vi "Get Loop Parameters.vi"(11 "error in (no error)":errorcluster) -> (4 "Sequence Type":T1, 6 "90Deg Pulse Sequence Array":T11[](array[typedef])=[{"Delay Settings"={"Delay d1"=100.0, "Delay d2"=2.0, "d1 Unit"=0, "d2 Unit"=0}, "Preliminary Settings"={"Nº of Scans (ns)"=3, "Pulse Frequency"=10000000.0}, "Pulse Settings"={"Duration Signal P1"=10.0, "Power Level"=1000, "Phase"=90, "P1 Units"=0}, "Acquisition Settings"={"Number Samples"=5000, "Time Between Points"=0.0, "Unit"=0}}, {"Delay Settings"={"Delay d1"=100.0, "Delay d2"=2.0, "d1 Unit"=0, "d2 Unit"=0}, "Preliminary Settings"={"Nº of Scans (ns)"=3, "Pulse Frequency"=10000000.0}, "Pulse Settings"={"Duration Signal P1"=20.0, "Power Level"=1000, "Phase"=90, "P1 Units"=0}, "Acquisition Settings"={"Number Samples"=5000, "Time Between Points"=0.0, "Unit"=0}}, {"Delay Settings"={"Delay d1"=100.0, "Delay d2"=2.0, "d1 Unit"=0, "d2 Unit"=0}, "Preliminary Settings"={"Nº of Scans (ns)"=3, "Pulse Frequency"=10000000.0}, "Pulse Settings"={"Duration Signal P1"=30.0, "Power Level"=1000, "Phase"=90, "P1 Units"=0}, "Acquisition Settings"={"Number Samples"=5000, "Time Between Points"=0.0, "Unit"=0}}, {"Delay Settings"={"Delay d1"=100.0, "Delay d2"=2.0, "d1 Unit"=0, "d2 Unit"=0}, "Preliminary Settings"={"Nº of Scans (ns)"=3, "Pulse Frequency"=10000000.0}, "Pulse Settings"={"Duration Signal P1"=40.0, "Power Level"=1000, "Phase"=90, "P1 Units"=0}, "Acquisition Settings"={"Number Samples"=5000, "Time Between Points"=0.0, "Unit"=0}}, {"Delay Settings"={"Delay d1"=100.0, "Delay d2"=2.0, "d1 Unit"=0, "d2 Unit"=0}, "Preliminary Settings"={"Nº of Scans (ns)"=3, "Pulse Frequency"=10000000.0}, "Pulse Settings"={"Duration Signal P1"=50.0, "Power Level"=1000, "Phase"=90, "P1 Units"=0}, "Acquisition Settings"={"Number Samples"=5000, "Time Between Points"=0.0, "Unit"=0}}, {"Delay Settings"={"Delay d1"=100.0, "Delay d2"=2.0, "d1 Unit"=0, "d2 Unit"=0}, "Preliminary Settings"={"Nº of Scans (ns)"=3, "Pulse Frequency"=10000000.0}, "Pulse Settings"={"Duration Signal P1"=60.0, "Power Level"=1000, "Phase"=90, "P1 Units"=0}, "Acquisition Settings"={"Number Samples"=5000, "Time Between Points"=0.0, "Unit"=0}}, {"Delay Settings"={"Delay d1"=100.0, "Delay d2"=2.0, "d1 Unit"=0, "d2 Unit"=0}, "Preliminary Settings"={"Nº of Scans (ns)"=3, "Pulse Frequency"=10000000.0}, "Pulse Settings"={"Duration Signal P1"=80.0, "Power Level"=1000, "Phase"=90, "P1 Units"=0}, "Acquisition Settings"={"Number Samples"=5000, "Time Between Points"=0.0, "Unit"=0}}, {"Delay Settings"={"Delay d1"=100.0, "Delay d2"=2.0, "d1 Unit"=0, "d2 Unit"=0}, "Preliminary Settings"={"Nº of Scans (ns)"=3, "Pulse Frequency"=10000000.0}, "Pulse Settings"={"Duration Signal P1"=90.0, "Power Level"=1000, "Phase"=90, "P1 Units"=0}, "Acquisition Settings"={"Number Samples"=5000, "Time Between Points"=0.0, "Unit"=0}}, {"Delay Settings"={"Delay d1"=100.0, "Delay d2"=2.0, "d1 Unit"=0, "d2 Unit"=0}, "Preliminary Settings"={"Nº of Scans (ns)"=3, "Pulse Frequency"=10000000.0}, "Pulse Settings"={"Duration Signal P1"=100.0, "Power Level"=1000, "Phase"=90, "P1 Units"=0}, "Acquisition Settings"={"Number Samples"=5000, "Time Between Points"=0.0, "Unit"=0}}, {"Delay Settings"={"Delay d1"=100.0, "Delay d2"=2.0, "d1 Unit"=0, "d2 Unit"=0}, "Preliminary Settings"={"Nº of Scans (ns)"=3, "Pulse Frequency"=9000000.0}, "Pulse Settings"={"Duration Signal P1"=10.0, "Power Level"=1000, "Phase"=90, "P1 Units"=0}, "Acquisition Settings"={"Number Samples"=5000, "Time Between Points"=0.0, "Unit"=0}}, {"Delay Settings"={"Delay d1"=100.0, "Delay d2"=2.0, "d1 Unit"=0, "d2 Unit"=0}, "Preliminary Settings"={"Nº of Scans (ns)"=3, "Pulse Frequency"=9000000.0}, "Pulse Settings"={"Duration Signal P1"=20.0, "Power Level"=1000, "Phase"=90, "P1 Units"=0}, "Acquisition Settings"={"Number Samples"=5000, "Time Between Points"=0.0, "Unit"=0}}, {"Delay Settings"={"Delay d1"=100.0, "Delay d2"=2.0, "d1 Unit"=0, "d2 Unit"=0}, "Preliminary Settings"={"Nº of Scans (ns)"=3, "Pulse Frequency"=9000000.0}, "Pulse Settings"={"Duration Signal P1"=30.0, "Power Level"=1000, "Phase"=90, "P1 Units"=0}, "Acquisition Settings"={"Number Samples"=5000, "Time Between Points"=0.0, "Unit"=0}}, {"Delay Settings"={"Delay d1"=100.0, "Delay d2"=2.0, "d1 Unit"=0, "d2 Unit"=0}, "Preliminary Settings"={"Nº of Scans (ns)"=3, "Pulse Frequency"=9000000.0}, "Pulse Settings"={"Duration Signal P1"=40.0, "Power Level"=1000, "Phase"=90, "P1 Units"=0}, "Acquisition Settings"={"Number Samples"=5000, "Time Between Points"=0.0, "Unit"=0}}, {"Delay Settings"={"Delay d1"=100.0, "Delay d2"=2.0, "d1 Unit"=0, "d2 Unit"=0}, "Preliminary Settings"={"Nº of Scans (ns)"=3, "Pulse Frequency"=9000000.0}, "Pulse Settings"={"Duration Signal P1"=50.0, "Power Level"=1000, "Phase"=90, "P1 Units"=0}, "Acquisition Settings"={"Number Samples"=5000, "Time Between Points"=0.0, "Unit"=0}}, {"Delay Settings"={"Delay d1"=100.0, "Delay d2"=2.0, "d1 Unit"=0, "d2 Unit"=0}, "Preliminary Settings"={"Nº of Scans (ns)"=3, "Pulse Frequency"=9000000.0}, "Pulse Settings"={"Duration Signal P1"=60.0, "Power Level"=1000, "Phase"=90, "P1 Units"=0}, "Acquisition Settings"={"Number Samples"=5000, "Time Between Points"=0.0, "Unit"=0}}, {"Delay Settings"={"Delay d1"=100.0, "Delay d2"=2.0, "d1 Unit"=0, "d2 Unit"=0}, "Preliminary Settings"={"Nº of Scans (ns)"=3, "Pulse Frequency"=9000000.0}, "Pulse Settings"={"Duration Signal P1"=80.0, "Power Level"=1000, "Phase"=90, "P1 Units"=0}, "Acquisition Settings"={"Number Samples"=5000, "Time Between Points"=0.0, "Unit"=0}}, {"Delay Settings"={"Delay d1"=100.0, "Delay d2"=2.0, "d1 Unit"=0, "d2 Unit"=0}, "Preliminary Settings"={"Nº of Scans (ns)"=3, "Pulse Frequency"=9000000.0}, "Pulse Settings"={"Duration Signal P1"=90.0, "Power Level"=1000, "Phase"=90, "P1 Units"=0}, "Acquisition Settings"={"Number Samples"=5000, "Time Between Points"=0.0, "Unit"=0}}, {"Delay Settings"={"Delay d1"=100.0, "Delay d2"=2.0, "d1 Unit"=0, "d2 Unit"=0}, "Preliminary Settings"={"Nº of Scans (ns)"=3, "Pulse Frequency"=9000000.0}, "Pulse Settings"={"Duration Signal P1"=100.0, "Power Level"=1000, "Phase"=90, "P1 Units"=0}, "Acquisition Settings"={"Number Samples"=5000, "Time Between Points"=0.0, "Unit"=0}}] {"Acquisition Settings"."Unit" items=["us", "ms"]; "Acquisition Settings"."Time Between Points" min=0.0 step=1.0; "Acquisition Settings"."Number Samples" step=1; "Pulse Settings"."P1 Units" items=["us", "ms"]; "Pulse Settings"."Phase" max=270 step=90; "Pulse Settings"."Power Level" max=1023 step=1; "Pulse Settings"."Duration Signal P1" min=0.0 step=1.0 format="%#_4g"; "Preliminary Settings"."Pulse Frequency" min=1.0 max=200000000.0 step=1000000.0 format="%^#_6e"; "Preliminary Settings"."Nº of Scans (ns)" step=1; "Delay Settings"."d2 Unit" items=["us", "ms"]; "Delay Settings"."d1 Unit" items=["us", "ms"]; "Delay Settings"."Delay d2" min=0.0 step=1.0 format="%#_4g"; "Delay Settings"."Delay d1" min=0.0 step=1.0 format="%#_4g"}, 8 "CPMG Pulse Sequence Array":T7[](array[typedef])=[{"Acquisition Settings"={"Number Samples"=5000, "Time Between Points"=0.0, "Unit"=0}, "Delay Settings"={"Delay d1"=100.0, "Delay d2"=2.0, "d1 Unit"=0, "d2 Unit"=0, "Delay d3"=100.0, "d3 Unit"=0, "Delay d4"=2.0, "d4 Unit"=0}, "Preliminary Settings"={"Nº of Scans (ns)"=3, "Pulse Frequency"=10000000.0, "Nº of Echoes (ne)"=3}, "Pulse Settings"={"Duration Signal P1"=10.0, "Power Level P1"=1000, "Phase P1"=90, "P1 Unit"=0, "Duration Signal P2"=10.0, "Power Level P2"=1000, "Phase P2"=90, "P2 Unit"=0}}, {"Acquisition Settings"={"Number Samples"=5000, "Time Between Points"=0.0, "Unit"=0}, "Delay Settings"={"Delay d1"=100.0, "Delay d2"=2.0, "d1 Unit"=0, "d2 Unit"=0, "Delay d3"=100.0, "d3 Unit"=0, "Delay d4"=2.0, "d4 Unit"=0}, "Preliminary Settings"={"Nº of Scans (ns)"=3, "Pulse Frequency"=10000000.0, "Nº of Echoes (ne)"=3}, "Pulse Settings"={"Duration Signal P1"=20.0, "Power Level P1"=1000, "Phase P1"=90, "P1 Unit"=0, "Duration Signal P2"=20.0, "Power Level P2"=1000, "Phase P2"=90, "P2 Unit"=0}}, {"Acquisition Settings"={"Number Samples"=5000, "Time Between Points"=0.0, "Unit"=0}, "Delay Settings"={"Delay d1"=100.0, "Delay d2"=2.0, "d1 Unit"=0, "d2 Unit"=0, "Delay d3"=100.0, "d3 Unit"=0, "Delay d4"=2.0, "d4 Unit"=0}, "Preliminary Settings"={"Nº of Scans (ns)"=3, "Pulse Frequency"=10000000.0, "Nº of Echoes (ne)"=3}, "Pulse Settings"={"Duration Signal P1"=30.0, "Power Level P1"=1000, "Phase P1"=90, "P1 Unit"=0, "Duration Signal P2"=30.0, "Power Level P2"=1000, "Phase P2"=90, "P2 Unit"=0}}, {"Acquisition Settings"={"Number Samples"=5000, "Time Between Points"=0.0, "Unit"=0}, "Delay Settings"={"Delay d1"=100.0, "Delay d2"=2.0, "d1 Unit"=0, "d2 Unit"=0, "Delay d3"=100.0, "d3 Unit"=0, "Delay d4"=2.0, "d4 Unit"=0}, "Preliminary Settings"={"Nº of Scans (ns)"=3, "Pulse Frequency"=10000000.0, "Nº of Echoes (ne)"=3}, "Pulse Settings"={"Duration Signal P1"=40.0, "Power Level P1"=1000, "Phase P1"=90, "P1 Unit"=0, "Duration Signal P2"=40.0, "Power Level P2"=1000, "Phase P2"=90, "P2 Unit"=0}}, {"Acquisition Settings"={"Number Samples"=5000, "Time Between Points"=0.0, "Unit"=0}, "Delay Settings"={"Delay d1"=100.0, "Delay d2"=2.0, "d1 Unit"=0, "d2 Unit"=0, "Delay d3"=100.0, "d3 Unit"=0, "Delay d4"=2.0, "d4 Unit"=0}, "Preliminary Settings"={"Nº of Scans (ns)"=3, "Pulse Frequency"=10000000.0, "Nº of Echoes (ne)"=3}, "Pulse Settings"={"Duration Signal P1"=50.0, "Power Level P1"=1000, "Phase P1"=90, "P1 Unit"=0, "Duration Signal P2"=50.0, "Power Level P2"=1000, "Phase P2"=90, "P2 Unit"=0}}, {"Acquisition Settings"={"Number Samples"=5000, "Time Between Points"=0.0, "Unit"=0}, "Delay Settings"={"Delay d1"=100.0, "Delay d2"=2.0, "d1 Unit"=0, "d2 Unit"=0, "Delay d3"=100.0, "d3 Unit"=0, "Delay d4"=2.0, "d4 Unit"=0}, "Preliminary Settings"={"Nº of Scans (ns)"=3, "Pulse Frequency"=10000000.0, "Nº of Echoes (ne)"=3}, "Pulse Settings"={"Duration Signal P1"=60.0, "Power Level P1"=1000, "Phase P1"=90, "P1 Unit"=0, "Duration Signal P2"=60.0, "Power Level P2"=1000, "Phase P2"=90, "P2 Unit"=0}}, {"Acquisition Settings"={"Number Samples"=5000, "Time Between Points"=0.0, "Unit"=0}, "Delay Settings"={"Delay d1"=100.0, "Delay d2"=2.0, "d1 Unit"=0, "d2 Unit"=0, "Delay d3"=100.0, "d3 Unit"=0, "Delay d4"=2.0, "d4 Unit"=0}, "Preliminary Settings"={"Nº of Scans (ns)"=3, "Pulse Frequency"=10000000.0, "Nº of Echoes (ne)"=3}, "Pulse Settings"={"Duration Signal P1"=80.0, "Power Level P1"=1000, "Phase P1"=90, "P1 Unit"=0, "Duration Signal P2"=80.0, "Power Level P2"=1000, "Phase P2"=90, "P2 Unit"=0}}, {"Acquisition Settings"={"Number Samples"=5000, "Time Between Points"=0.0, "Unit"=0}, "Delay Settings"={"Delay d1"=100.0, "Delay d2"=2.0, "d1 Unit"=0, "d2 Unit"=0, "Delay d3"=100.0, "d3 Unit"=0, "Delay d4"=2.0, "d4 Unit"=0}, "Preliminary Settings"={"Nº of Scans (ns)"=3, "Pulse Frequency"=10000000.0, "Nº of Echoes (ne)"=3}, "Pulse Settings"={"Duration Signal P1"=90.0, "Power Level P1"=1000, "Phase P1"=90, "P1 Unit"=0, "Duration Signal P2"=90.0, "Power Level P2"=1000, "Phase P2"=90, "P2 Unit"=0}}, {"Acquisition Settings"={"Number Samples"=5000, "Time Between Points"=0.0, "Unit"=0}, "Delay Settings"={"Delay d1"=100.0, "Delay d2"=2.0, "d1 Unit"=0, "d2 Unit"=0, "Delay d3"=100.0, "d3 Unit"=0, "Delay d4"=2.0, "d4 Unit"=0}, "Preliminary Settings"={"Nº of Scans (ns)"=3, "Pulse Frequency"=10000000.0, "Nº of Echoes (ne)"=3}, "Pulse Settings"={"Duration Signal P1"=100.0, "Power Level P1"=1000, "Phase P1"=90, "P1 Unit"=0, "Duration Signal P2"=100.0, "Power Level P2"=1000, "Phase P2"=90, "P2 Unit"=0}}, {"Acquisition Settings"={"Number Samples"=5000, "Time Between Points"=0.0, "Unit"=0}, "Delay Settings"={"Delay d1"=100.0, "Delay d2"=2.0, "d1 Unit"=0, "d2 Unit"=0, "Delay d3"=100.0, "d3 Unit"=0, "Delay d4"=2.0, "d4 Unit"=0}, "Preliminary Settings"={"Nº of Scans (ns)"=3, "Pulse Frequency"=9000000.0, "Nº of Echoes (ne)"=3}, "Pulse Settings"={"Duration Signal P1"=10.0, "Power Level P1"=1000, "Phase P1"=90, "P1 Unit"=0, "Duration Signal P2"=10.0, "Power Level P2"=1000, "Phase P2"=90, "P2 Unit"=0}}, {"Acquisition Settings"={"Number Samples"=5000, "Time Between Points"=0.0, "Unit"=0}, "Delay Settings"={"Delay d1"=100.0, "Delay d2"=2.0, "d1 Unit"=0, "d2 Unit"=0, "Delay d3"=100.0, "d3 Unit"=0, "Delay d4"=2.0, "d4 Unit"=0}, "Preliminary Settings"={"Nº of Scans (ns)"=3, "Pulse Frequency"=9000000.0, "Nº of Echoes (ne)"=3}, "Pulse Settings"={"Duration Signal P1"=20.0, "Power Level P1"=1000, "Phase P1"=90, "P1 Unit"=0, "Duration Signal P2"=20.0, "Power Level P2"=1000, "Phase P2"=90, "P2 Unit"=0}}, {"Acquisition Settings"={"Number Samples"=5000, "Time Between Points"=0.0, "Unit"=0}, "Delay Settings"={"Delay d1"=100.0, "Delay d2"=2.0, "d1 Unit"=0, "d2 Unit"=0, "Delay d3"=100.0, "d3 Unit"=0, "Delay d4"=2.0, "d4 Unit"=0}, "Preliminary Settings"={"Nº of Scans (ns)"=3, "Pulse Frequency"=9000000.0, "Nº of Echoes (ne)"=3}, "Pulse Settings"={"Duration Signal P1"=30.0, "Power Level P1"=1000, "Phase P1"=90, "P1 Unit"=0, "Duration Signal P2"=30.0, "Power Level P2"=1000, "Phase P2"=90, "P2 Unit"=0}}, {"Acquisition Settings"={"Number Samples"=5000, "Time Between Points"=0.0, "Unit"=0}, "Delay Settings"={"Delay d1"=100.0, "Delay d2"=2.0, "d1 Unit"=0, "d2 Unit"=0, "Delay d3"=100.0, "d3 Unit"=0, "Delay d4"=2.0, "d4 Unit"=0}, "Preliminary Settings"={"Nº of Scans (ns)"=3, "Pulse Frequency"=9000000.0, "Nº of Echoes (ne)"=3}, "Pulse Settings"={"Duration Signal P1"=40.0, "Power Level P1"=1000, "Phase P1"=90, "P1 Unit"=0, "Duration Signal P2"=40.0, "Power Level P2"=1000, "Phase P2"=90, "P2 Unit"=0}}, {"Acquisition Settings"={"Number Samples"=5000, "Time Between Points"=0.0, "Unit"=0}, "Delay Settings"={"Delay d1"=100.0, "Delay d2"=2.0, "d1 Unit"=0, "d2 Unit"=0, "Delay d3"=100.0, "d3 Unit"=0, "Delay d4"=2.0, "d4 Unit"=0}, "Preliminary Settings"={"Nº of Scans (ns)"=3, "Pulse Frequency"=9000000.0, "Nº of Echoes (ne)"=3}, "Pulse Settings"={"Duration Signal P1"=50.0, "Power Level P1"=1000, "Phase P1"=90, "P1 Unit"=0, "Duration Signal P2"=50.0, "Power Level P2"=1000, "Phase P2"=90, "P2 Unit"=0}}, {"Acquisition Settings"={"Number Samples"=5000, "Time Between Points"=0.0, "Unit"=0}, "Delay Settings"={"Delay d1"=100.0, "Delay d2"=2.0, "d1 Unit"=0, "d2 Unit"=0, "Delay d3"=100.0, "d3 Unit"=0, "Delay d4"=2.0, "d4 Unit"=0}, "Preliminary Settings"={"Nº of Scans (ns)"=3, "Pulse Frequency"=9000000.0, "Nº of Echoes (ne)"=3}, "Pulse Settings"={"Duration Signal P1"=60.0, "Power Level P1"=1000, "Phase P1"=90, "P1 Unit"=0, "Duration Signal P2"=60.0, "Power Level P2"=1000, "Phase P2"=90, "P2 Unit"=0}}, {"Acquisition Settings"={"Number Samples"=5000, "Time Between Points"=0.0, "Unit"=0}, "Delay Settings"={"Delay d1"=100.0, "Delay d2"=2.0, "d1 Unit"=0, "d2 Unit"=0, "Delay d3"=100.0, "d3 Unit"=0, "Delay d4"=2.0, "d4 Unit"=0}, "Preliminary Settings"={"Nº of Scans (ns)"=3, "Pulse Frequency"=9000000.0, "Nº of Echoes (ne)"=3}, "Pulse Settings"={"Duration Signal P1"=80.0, "Power Level P1"=1000, "Phase P1"=90, "P1 Unit"=0, "Duration Signal P2"=80.0, "Power Level P2"=1000, "Phase P2"=90, "P2 Unit"=0}}, {"Acquisition Settings"={"Number Samples"=5000, "Time Between Points"=0.0, "Unit"=0}, "Delay Settings"={"Delay d1"=100.0, "Delay d2"=2.0, "d1 Unit"=0, "d2 Unit"=0, "Delay d3"=100.0, "d3 Unit"=0, "Delay d4"=2.0, "d4 Unit"=0}, "Preliminary Settings"={"Nº of Scans (ns)"=3, "Pulse Frequency"=9000000.0, "Nº of Echoes (ne)"=3}, "Pulse Settings"={"Duration Signal P1"=90.0, "Power Level P1"=1000, "Phase P1"=90, "P1 Unit"=0, "Duration Signal P2"=90.0, "Power Level P2"=1000, "Phase P2"=90, "P2 Unit"=0}}, {"Acquisition Settings"={"Number Samples"=5000, "Time Between Points"=0.0, "Unit"=0}, "Delay Settings"={"Delay d1"=100.0, "Delay d2"=2.0, "d1 Unit"=0, "d2 Unit"=0, "Delay d3"=100.0, "d3 Unit"=0, "Delay d4"=2.0, "d4 Unit"=0}, "Preliminary Settings"={"Nº of Scans (ns)"=3, "Pulse Frequency"=9000000.0, "Nº of Echoes (ne)"=3}, "Pulse Settings"={"Duration Signal P1"=100.0, "Power Level P1"=1000, "Phase P1"=90, "P1 Unit"=0, "Duration Signal P2"=100.0, "Power Level P2"=1000, "Phase P2"=90, "P2 Unit"=0}}] {"Pulse Settings"."P2 Unit" items=["us", "ms"]; "Pulse Settings"."Phase P2" max=270 step=90; "Pulse Settings"."Power Level P2" max=1023 step=1; "Pulse Settings"."Duration Signal P2" min=0.0 step=1.0 format="%#_4g"; "Pulse Settings"."P1 Unit" items=["us", "ms"]; "Pulse Settings"."Phase P1" max=270 step=90; "Pulse Settings"."Power Level P1" max=1023 step=1; "Pulse Settings"."Duration Signal P1" min=0.0 step=1.0 format="%#_4g"; "Preliminary Settings"."Nº of Echoes (ne)" step=1; "Preliminary Settings"."Pulse Frequency" min=1.0 max=200000000.0 step=1000000.0 format="%^#_6e"; "Preliminary Settings"."Nº of Scans (ns)" step=1; "Delay Settings"."d4 Unit" items=["us", "ms"]; "Delay Settings"."Delay d4" min=0.0 step=1.0 format="%#_4g"; "Delay Settings"."d3 Unit" items=["us", "ms"]; "Delay Settings"."Delay d3" min=0.0 step=1.0 format="%#_4g"; "Delay Settings"."d2 Unit" items=["us", "ms"]; "Delay Settings"."d1 Unit" items=["us", "ms"]; "Delay Settings"."Delay d2" min=0.0 step=1.0 format="%#_4g"; "Delay Settings"."Delay d1" min=0.0 step=1.0 format="%#_4g"; "Acquisition Settings"."Unit" items=["us", "ms"]; "Acquisition Settings"."Time Between Points" min=0.0 step=1.0; "Acquisition Settings"."Number Samples" step=1}, 10 "T1 Pulse Sequence Array":T2[](array[typedef])=[{"Preliminary Settings"={"Nº of Scans (ns)"=3, "Pulse Frequency"=10000000.0, "Nº of Vd"=3}, "Pulse Settings"={"Duration Signal P2"=10.0, "Power Level P2"=1000, "Phase P2"=90, "P2 Unit"=0, "Duration Signal P1"=10.0, "Power Level P1"=1000, "Phase P1"=90, "P1 Unit"=0}, "Acquisition Settings"={"Number Samples"=5000, "Time Between Points"=0.0, "Unit"=0}, "Delay Settings"={"Delay d1"=100.0, "Delay d2"=2.0, "d1 Unit"=0, "d2 Unit"=0, "Delay d30"=0.0, "d30 Unit"=0, "Vd Unit"=0, "Vd Values"="Automatic"}}, {"Preliminary Settings"={"Nº of Scans (ns)"=3, "Pulse Frequency"=10000000.0, "Nº of Vd"=3}, "Pulse Settings"={"Duration Signal P2"=20.0, "Power Level P2"=1000, "Phase P2"=90, "P2 Unit"=0, "Duration Signal P1"=20.0, "Power Level P1"=1000, "Phase P1"=90, "P1 Unit"=0}, "Acquisition Settings"={"Number Samples"=5000, "Time Between Points"=0.0, "Unit"=0}, "Delay Settings"={"Delay d1"=100.0, "Delay d2"=2.0, "d1 Unit"=0, "d2 Unit"=0, "Delay d30"=0.0, "d30 Unit"=0, "Vd Unit"=0, "Vd Values"="Automatic"}}, {"Preliminary Settings"={"Nº of Scans (ns)"=3, "Pulse Frequency"=10000000.0, "Nº of Vd"=3}, "Pulse Settings"={"Duration Signal P2"=30.0, "Power Level P2"=1000, "Phase P2"=90, "P2 Unit"=0, "Duration Signal P1"=30.0, "Power Level P1"=1000, "Phase P1"=90, "P1 Unit"=0}, "Acquisition Settings"={"Number Samples"=5000, "Time Between Points"=0.0, "Unit"=0}, "Delay Settings"={"Delay d1"=100.0, "Delay d2"=2.0, "d1 Unit"=0, "d2 Unit"=0, "Delay d30"=0.0, "d30 Unit"=0, "Vd Unit"=0, "Vd Values"="Automatic"}}, {"Preliminary Settings"={"Nº of Scans (ns)"=3, "Pulse Frequency"=10000000.0, "Nº of Vd"=3}, "Pulse Settings"={"Duration Signal P2"=40.0, "Power Level P2"=1000, "Phase P2"=90, "P2 Unit"=0, "Duration Signal P1"=40.0, "Power Level P1"=1000, "Phase P1"=90, "P1 Unit"=0}, "Acquisition Settings"={"Number Samples"=5000, "Time Between Points"=1.0, "Unit"=0}, "Delay Settings"={"Delay d1"=100.0, "Delay d2"=2.0, "d1 Unit"=0, "d2 Unit"=0, "Delay d30"=0.0, "d30 Unit"=0, "Vd Unit"=0, "Vd Values"="Automatic"}}, {"Preliminary Settings"={"Nº of Scans (ns)"=3, "Pulse Frequency"=10000000.0, "Nº of Vd"=3}, "Pulse Settings"={"Duration Signal P2"=50.0, "Power Level P2"=1000, "Phase P2"=90, "P2 Unit"=0, "Duration Signal P1"=50.0, "Power Level P1"=1000, "Phase P1"=90, "P1 Unit"=0}, "Acquisition Settings"={"Number Samples"=5000, "Time Between Points"=0.0, "Unit"=0}, "Delay Settings"={"Delay d1"=100.0, "Delay d2"=2.0, "d1 Unit"=0, "d2 Unit"=0, "Delay d30"=0.0, "d30 Unit"=0, "Vd Unit"=0, "Vd Values"="Automatic"}}, {"Preliminary Settings"={"Nº of Scans (ns)"=3, "Pulse Frequency"=10000000.0, "Nº of Vd"=3}, "Pulse Settings"={"Duration Signal P2"=60.0, "Power Level P2"=1000, "Phase P2"=90, "P2 Unit"=0, "Duration Signal P1"=60.0, "Power Level P1"=1000, "Phase P1"=90, "P1 Unit"=0}, "Acquisition Settings"={"Number Samples"=5000, "Time Between Points"=0.0, "Unit"=0}, "Delay Settings"={"Delay d1"=100.0, "Delay d2"=2.0, "d1 Unit"=0, "d2 Unit"=0, "Delay d30"=0.0, "d30 Unit"=0, "Vd Unit"=0, "Vd Values"="Automatic"}}, {"Preliminary Settings"={"Nº of Scans (ns)"=3, "Pulse Frequency"=10000000.0, "Nº of Vd"=3}, "Pulse Settings"={"Duration Signal P2"=80.0, "Power Level P2"=1000, "Phase P2"=90, "P2 Unit"=0, "Duration Signal P1"=80.0, "Power Level P1"=1000, "Phase P1"=90, "P1 Unit"=0}, "Acquisition Settings"={"Number Samples"=5000, "Time Between Points"=1.0, "Unit"=0}, "Delay Settings"={"Delay d1"=100.0, "Delay d2"=2.0, "d1 Unit"=0, "d2 Unit"=0, "Delay d30"=0.0, "d30 Unit"=0, "Vd Unit"=0, "Vd Values"="Automatic"}}, {"Preliminary Settings"={"Nº of Scans (ns)"=3, "Pulse Frequency"=10000000.0, "Nº of Vd"=3}, "Pulse Settings"={"Duration Signal P2"=90.0, "Power Level P2"=1000, "Phase P2"=90, "P2 Unit"=0, "Duration Signal P1"=90.0, "Power Level P1"=1000, "Phase P1"=90, "P1 Unit"=0}, "Acquisition Settings"={"Number Samples"=5000, "Time Between Points"=0.0, "Unit"=0}, "Delay Settings"={"Delay d1"=100.0, "Delay d2"=2.0, "d1 Unit"=0, "d2 Unit"=0, "Delay d30"=0.0, "d30 Unit"=0, "Vd Unit"=0, "Vd Values"="Automatic"}}, {"Preliminary Settings"={"Nº of Scans (ns)"=3, "Pulse Frequency"=10000000.0, "Nº of Vd"=3}, "Pulse Settings"={"Duration Signal P2"=100.0, "Power Level P2"=1000, "Phase P2"=90, "P2 Unit"=0, "Duration Signal P1"=100.0, "Power Level P1"=1000, "Phase P1"=90, "P1 Unit"=0}, "Acquisition Settings"={"Number Samples"=5000, "Time Between Points"=1.0, "Unit"=0}, "Delay Settings"={"Delay d1"=100.0, "Delay d2"=2.0, "d1 Unit"=0, "d2 Unit"=0, "Delay d30"=0.0, "d30 Unit"=0, "Vd Unit"=0, "Vd Values"="Automatic"}}, {"Preliminary Settings"={"Nº of Scans (ns)"=3, "Pulse Frequency"=9000000.0, "Nº of Vd"=3}, "Pulse Settings"={"Duration Signal P2"=10.0, "Power Level P2"=1000, "Phase P2"=90, "P2 Unit"=0, "Duration Signal P1"=10.0, "Power Level P1"=1000, "Phase P1"=90, "P1 Unit"=0}, "Acquisition Settings"={"Number Samples"=5000, "Time Between Points"=20.0, "Unit"=0}, "Delay Settings"={"Delay d1"=100.0, "Delay d2"=2.0, "d1 Unit"=0, "d2 Unit"=0, "Delay d30"=0.0, "d30 Unit"=0, "Vd Unit"=0, "Vd Values"="Automatic"}}, {"Preliminary Settings"={"Nº of Scans (ns)"=3, "Pulse Frequency"=9000000.0, "Nº of Vd"=3}, "Pulse Settings"={"Duration Signal P2"=20.0, "Power Level P2"=1000, "Phase P2"=90, "P2 Unit"=0, "Duration Signal P1"=20.0, "Power Level P1"=1000, "Phase P1"=90, "P1 Unit"=0}, "Acquisition Settings"={"Number Samples"=5000, "Time Between Points"=0.0, "Unit"=0}, "Delay Settings"={"Delay d1"=100.0, "Delay d2"=2.0, "d1 Unit"=0, "d2 Unit"=0, "Delay d30"=0.0, "d30 Unit"=0, "Vd Unit"=0, "Vd Values"="Automatic"}}, {"Preliminary Settings"={"Nº of Scans (ns)"=3, "Pulse Frequency"=9000000.0, "Nº of Vd"=3}, "Pulse Settings"={"Duration Signal P2"=30.0, "Power Level P2"=1000, "Phase P2"=90, "P2 Unit"=0, "Duration Signal P1"=30.0, "Power Level P1"=1000, "Phase P1"=90, "P1 Unit"=0}, "Acquisition Settings"={"Number Samples"=5000, "Time Between Points"=0.0, "Unit"=0}, "Delay Settings"={"Delay d1"=100.0, "Delay d2"=2.0, "d1 Unit"=0, "d2 Unit"=0, "Delay d30"=0.0, "d30 Unit"=0, "Vd Unit"=0, "Vd Values"="Automatic"}}, {"Preliminary Settings"={"Nº of Scans (ns)"=3, "Pulse Frequency"=9000000.0, "Nº of Vd"=3}, "Pulse Settings"={"Duration Signal P2"=40.0, "Power Level P2"=1000, "Phase P2"=90, "P2 Unit"=0, "Duration Signal P1"=40.0, "Power Level P1"=1000, "Phase P1"=90, "P1 Unit"=0}, "Acquisition Settings"={"Number Samples"=5000, "Time Between Points"=20.0, "Unit"=0}, "Delay Settings"={"Delay d1"=100.0, "Delay d2"=2.0, "d1 Unit"=0, "d2 Unit"=0, "Delay d30"=0.0, "d30 Unit"=0, "Vd Unit"=0, "Vd Values"="Automatic"}}, {"Preliminary Settings"={"Nº of Scans (ns)"=3, "Pulse Frequency"=9000000.0, "Nº of Vd"=3}, "Pulse Settings"={"Duration Signal P2"=50.0, "Power Level P2"=1000, "Phase P2"=90, "P2 Unit"=0, "Duration Signal P1"=50.0, "Power Level P1"=1000, "Phase P1"=90, "P1 Unit"=0}, "Acquisition Settings"={"Number Samples"=5000, "Time Between Points"=0.0, "Unit"=0}, "Delay Settings"={"Delay d1"=100.0, "Delay d2"=2.0, "d1 Unit"=0, "d2 Unit"=0, "Delay d30"=0.0, "d30 Unit"=0, "Vd Unit"=0, "Vd Values"="Automatic"}}, {"Preliminary Settings"={"Nº of Scans (ns)"=3, "Pulse Frequency"=9000000.0, "Nº of Vd"=3}, "Pulse Settings"={"Duration Signal P2"=60.0, "Power Level P2"=1000, "Phase P2"=90, "P2 Unit"=0, "Duration Signal P1"=60.0, "Power Level P1"=1000, "Phase P1"=90, "P1 Unit"=0}, "Acquisition Settings"={"Number Samples"=5000, "Time Between Points"=0.0, "Unit"=0}, "Delay Settings"={"Delay d1"=100.0, "Delay d2"=2.0, "d1 Unit"=0, "d2 Unit"=0, "Delay d30"=0.0, "d30 Unit"=0, "Vd Unit"=0, "Vd Values"="Automatic"}}, {"Preliminary Settings"={"Nº of Scans (ns)"=3, "Pulse Frequency"=9000000.0, "Nº of Vd"=3}, "Pulse Settings"={"Duration Signal P2"=80.0, "Power Level P2"=1000, "Phase P2"=90, "P2 Unit"=0, "Duration Signal P1"=80.0, "Power Level P1"=1000, "Phase P1"=90, "P1 Unit"=0}, "Acquisition Settings"={"Number Samples"=5000, "Time Between Points"=0.0, "Unit"=0}, "Delay Settings"={"Delay d1"=100.0, "Delay d2"=2.0, "d1 Unit"=0, "d2 Unit"=0, "Delay d30"=0.0, "d30 Unit"=0, "Vd Unit"=0, "Vd Values"="Automatic"}}, {"Preliminary Settings"={"Nº of Scans (ns)"=3, "Pulse Frequency"=9000000.0, "Nº of Vd"=3}, "Pulse Settings"={"Duration Signal P2"=90.0, "Power Level P2"=1000, "Phase P2"=90, "P2 Unit"=0, "Duration Signal P1"=90.0, "Power Level P1"=1000, "Phase P1"=90, "P1 Unit"=0}, "Acquisition Settings"={"Number Samples"=5000, "Time Between Points"=20.0, "Unit"=0}, "Delay Settings"={"Delay d1"=100.0, "Delay d2"=2.0, "d1 Unit"=0, "d2 Unit"=0, "Delay d30"=0.0, "d30 Unit"=0, "Vd Unit"=0, "Vd Values"="Automatic"}}, {"Preliminary Settings"={"Nº of Scans (ns)"=3, "Pulse Frequency"=9000000.0, "Nº of Vd"=3}, "Pulse Settings"={"Duration Signal P2"=100.0, "Power Level P2"=1000, "Phase P2"=90, "P2 Unit"=0, "Duration Signal P1"=100.0, "Power Level P1"=1000, "Phase P1"=90, "P1 Unit"=0}, "Acquisition Settings"={"Number Samples"=5000, "Time Between Points"=20.0, "Unit"=0}, "Delay Settings"={"Delay d1"=100.0, "Delay d2"=2.0, "d1 Unit"=0, "d2 Unit"=0, "Delay d30"=0.0, "d30 Unit"=0, "Vd Unit"=0, "Vd Values"="Automatic"}}] {"Delay Settings"."Vd Unit" items=["us", "ms"]; "Delay Settings"."d30 Unit" items=["us", "ms"]; "Delay Settings"."Delay d30" min=0.0 step=1.0; "Delay Settings"."d2 Unit" items=["us", "ms"]; "Delay Settings"."d1 Unit" items=["us", "ms"]; "Delay Settings"."Delay d2" min=0.0 step=1.0 format="%#_4g"; "Delay Settings"."Delay d1" min=0.0 step=1.0 format="%#_4g"; "Acquisition Settings"."Unit" items=["us", "ms"]; "Acquisition Settings"."Time Between Points" min=0.0 step=1.0; "Acquisition Settings"."Number Samples" step=1; "Pulse Settings"."P1 Unit" items=["us", "ms"]; "Pulse Settings"."Phase P1" max=270 step=90; "Pulse Settings"."Power Level P1" max=1023 step=1; "Pulse Settings"."Duration Signal P1" min=0.0 step=1.0 format="%#_4g"; "Pulse Settings"."P2 Unit" items=["us", "ms"]; "Pulse Settings"."Phase P2" max=270 step=90; "Pulse Settings"."Power Level P2" max=1023 step=1; "Pulse Settings"."Duration Signal P2" min=0.0 step=1.0 format="%#_4g"; "Preliminary Settings"."Nº of Vd" step=1; "Preliminary Settings"."Pulse Frequency" min=1.0 max=200000000.0 step=1000000.0 format="%^#_6e"; "Preliminary Settings"."Nº of Scans (ns)" step=1}, 12 "90Deg path array":path[](array[path]), 13 "CPMG Path array":path[](array[path]), 14 "T1 path array":path[](array[path]), 15 "error out":errorcluster)   [LabVIEW 2011]
uses:
  Controls/Full_90 Degree Pulse Settings.ctl
  Controls/90D_Delay Settings.ctl
  Controls/90D_Preliminary Settings.ctl
  Controls/90D_Pulse Settings.ctl
  Controls/Acquisition Settings.ctl
  Controls/Full_CPMG Degree Pulse Settings.ctl
  Controls/CPMG_Delay Settings.ctl
  Controls/CPMG_Preliminary Settings.ctl
  Controls/CPMG_Pulse Settings.ctl
  Controls/Full_T1 Degree Pulse Settings.ctl
  Controls/T1_Preliminary Settings.ctl
  Controls/T1_Pulse Settings.ctl
  Controls/T1_Delay Settings.ctl
  Controls/NMR Pulse Sequence Type.ctl
  <vilib>/Utility/file.llb/Read From Spreadsheet File (string).vi
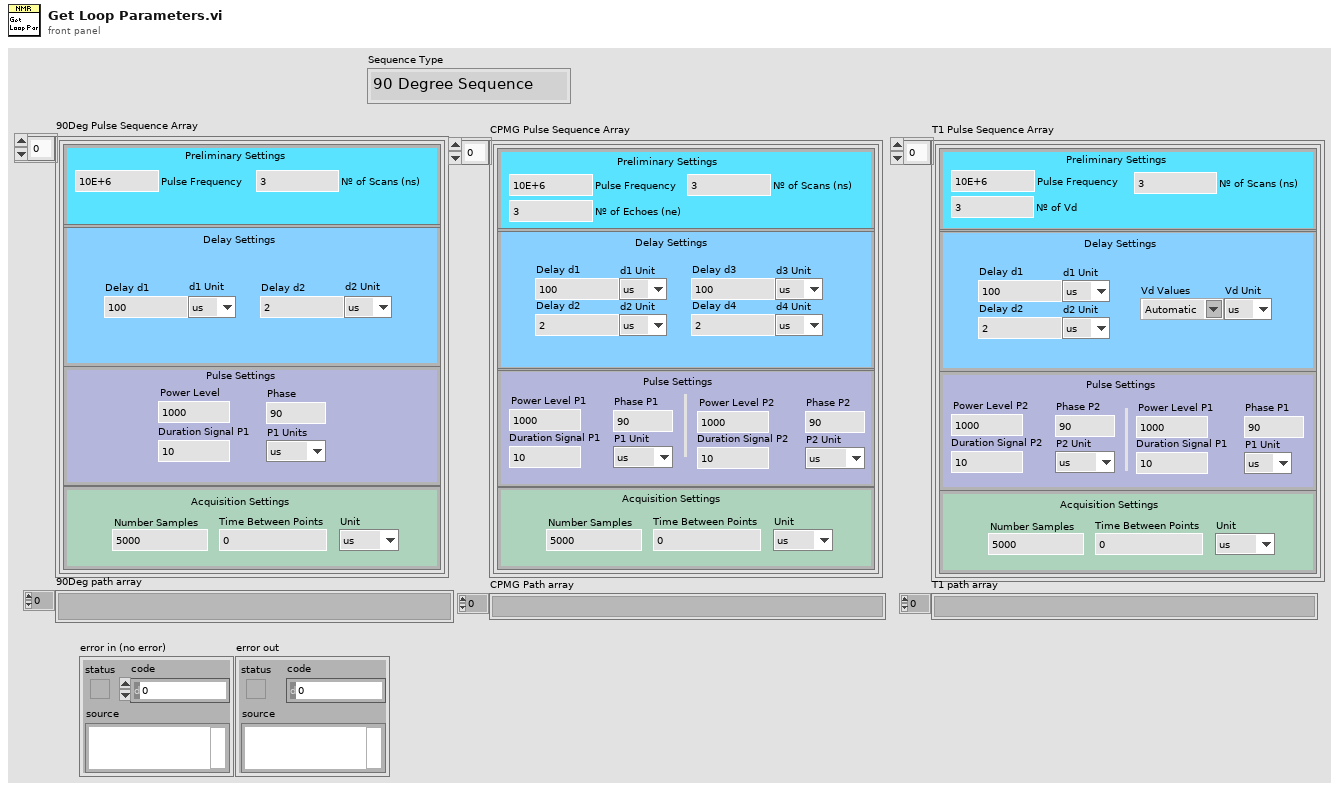
[diagram p1: front panel]
types:
  T1 = typedef "NMR Pulse Sequence Type.ctl" = enum16{"90 Degree Sequence", "CPMG Pulse Sequence", "T1 Pulse Sequence"}
  T2 = typedef "Full_T1 Degree Pulse Settings.ctl" = cluster{"Preliminary Settings":T3, "Pulse Settings":T4, "Acquisition Settings":T5, "Delay Settings":T6}
  T3 = typedef "T1_Preliminary Settings.ctl" = cluster{"Nº of Scans (ns)":u16, "Pulse Frequency":dbl, "Nº of Vd":u16}
  T4 = typedef "T1_Pulse Settings.ctl" = cluster{"Duration Signal P2":dbl, "Power Level P2":u16, "Phase P2":u16, "P2 Unit":u8, "Duration Signal P1":dbl, "Power Level P1":u16, "Phase P1":u16, "P1 Unit":u8}
  T5 = typedef "Acquisition Settings.ctl" = cluster{"Number Samples":u16, "Time Between Points":dbl, "Unit":u8}
  T6 = typedef "T1_Delay Settings.ctl" = cluster{"Delay d1":dbl, "Delay d2":dbl, "d1 Unit":u8, "d2 Unit":u8, "Delay d30":dbl, "d30 Unit":u8, "Vd Unit":u8, "Vd Values":string}
  T7 = typedef "Full_CPMG Degree Pulse Settings.ctl" = cluster{"Acquisition Settings":T5, "Delay Settings":T8, "Preliminary Settings":T9, "Pulse Settings":T10}
  T8 = typedef "CPMG_Delay Settings.ctl" = cluster{"Delay d1":dbl, "Delay d2":dbl, "d1 Unit":u8, "d2 Unit":u8, "Delay d3":dbl, "d3 Unit":u8, "Delay d4":dbl, "d4 Unit":u8}
  T9 = typedef "CPMG_Preliminary Settings.ctl" = cluster{"Nº of Scans (ns)":u16, "Pulse Frequency":dbl, "Nº of Echoes (ne)":u16}
  T10 = typedef "CPMG_Pulse Settings.ctl" = cluster{"Duration Signal P1":dbl, "Power Level P1":u16, "Phase P1":u16, "P1 Unit":u8, "Duration Signal P2":dbl, "Power Level P2":u16, "Phase P2":u16, "P2 Unit":u8}
  T11 = typedef "Full_90 Degree Pulse Settings.ctl" = cluster{"Delay Settings":T12, "Preliminary Settings":T13, "Pulse Settings":T14, "Acquisition Settings":T5}
  T12 = typedef "90D_Delay Settings.ctl" = cluster{"Delay d1":dbl, "Delay d2":dbl, "d1 Unit":u8, "d2 Unit":u8}
  T13 = typedef "90D_Preliminary Settings.ctl" = cluster{"Nº of Scans (ns)":u16, "Pulse Frequency":dbl}
  T14 = typedef "90D_Pulse Settings.ctl" = cluster{"Duration Signal P1":dbl, "Power Level":u16, "Phase":u16, "P1 Units":u8}
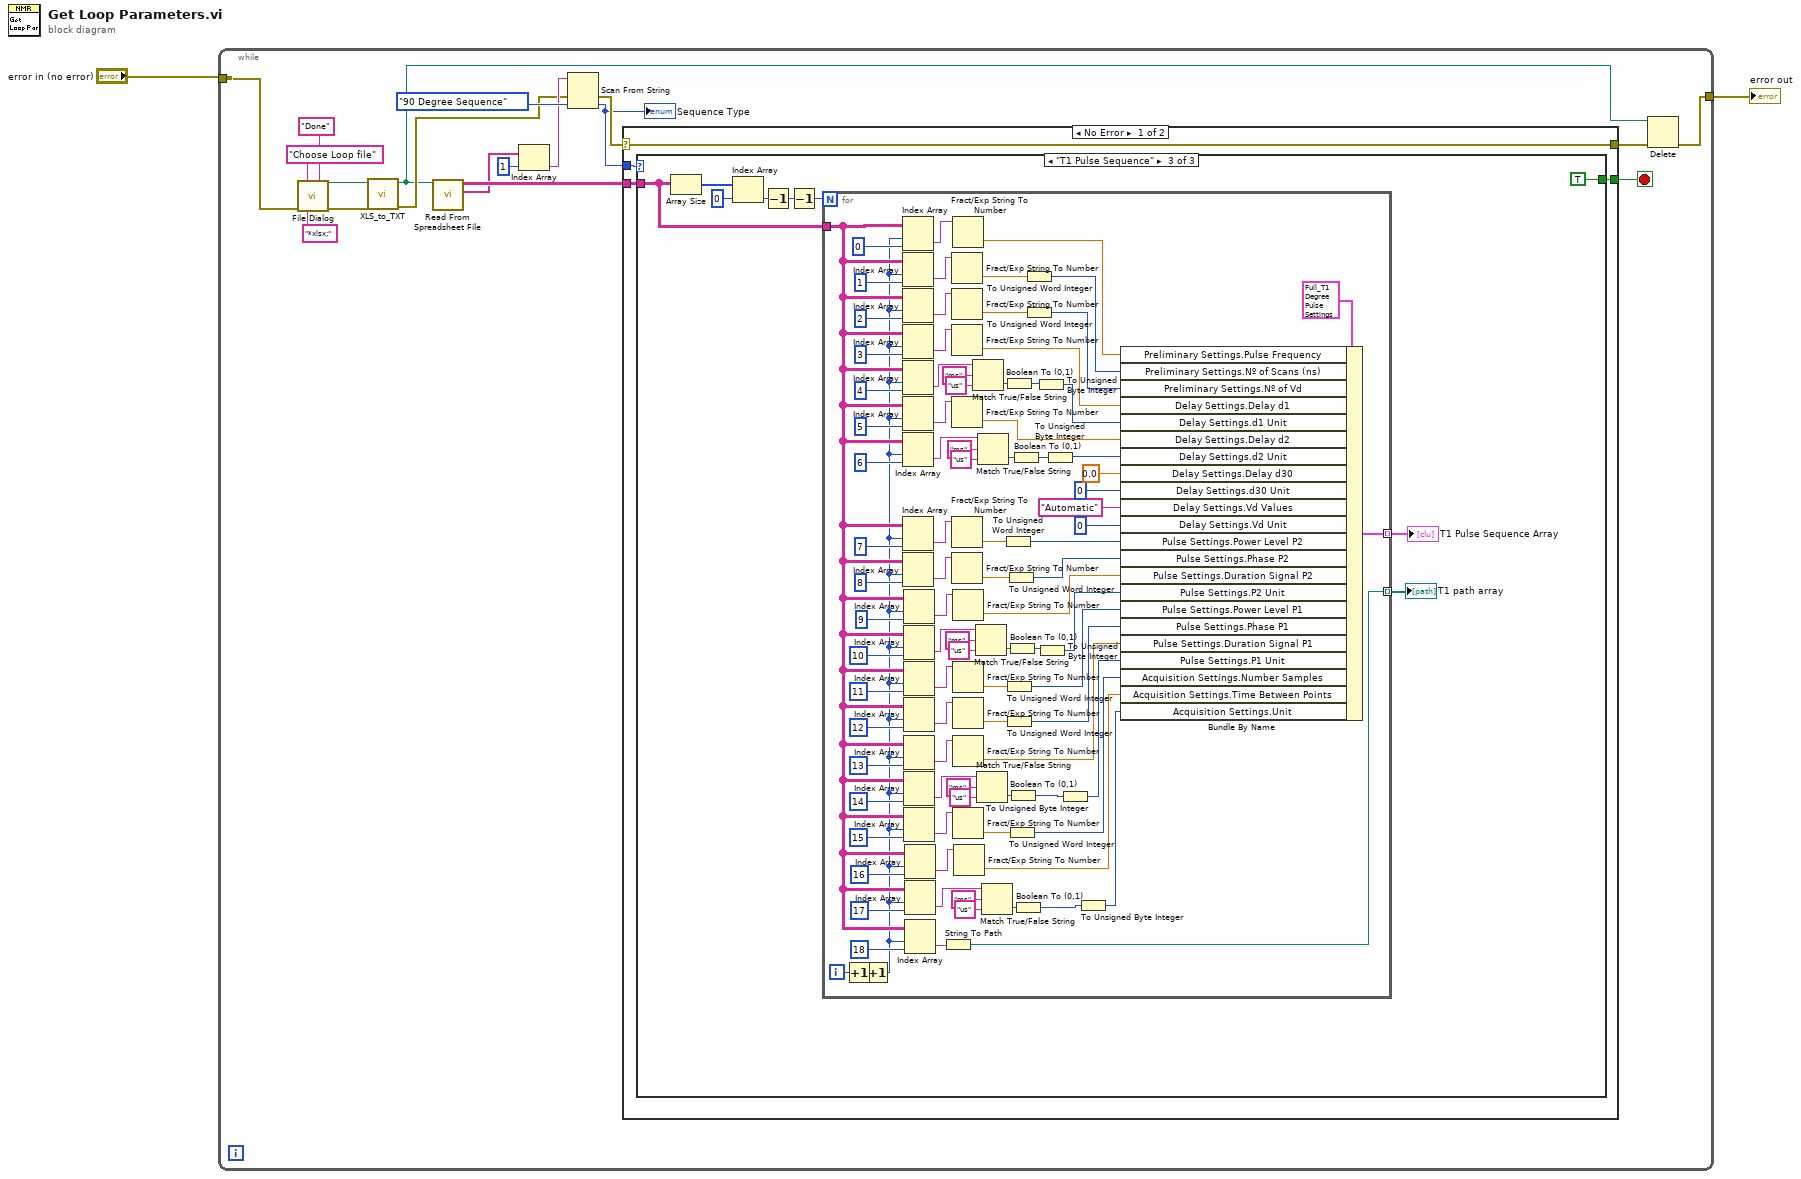
[diagram p0: block diagram]
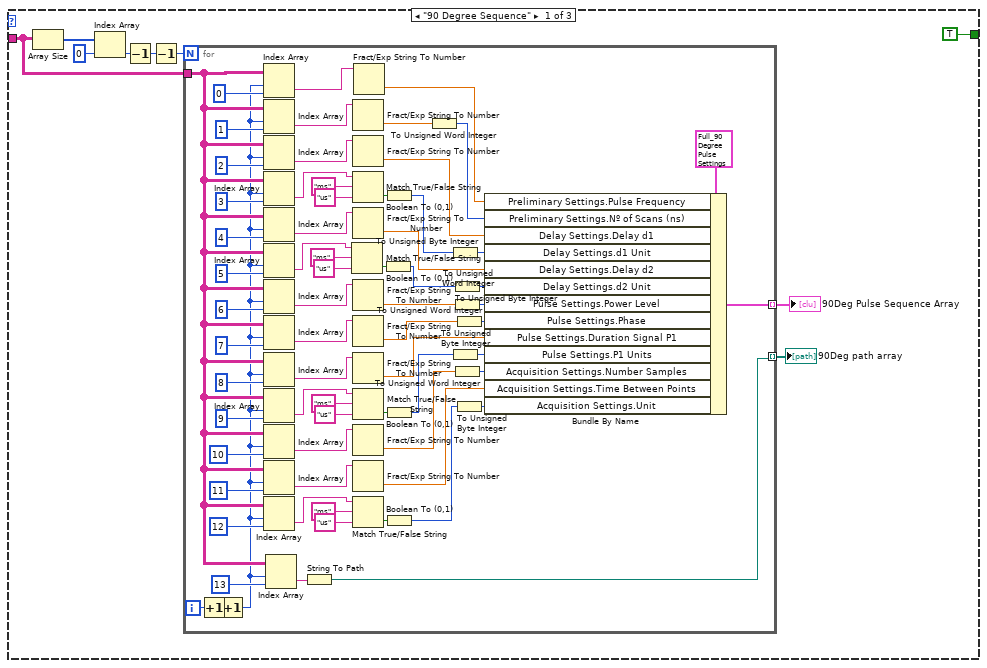
[diagram p2: hidden frame]
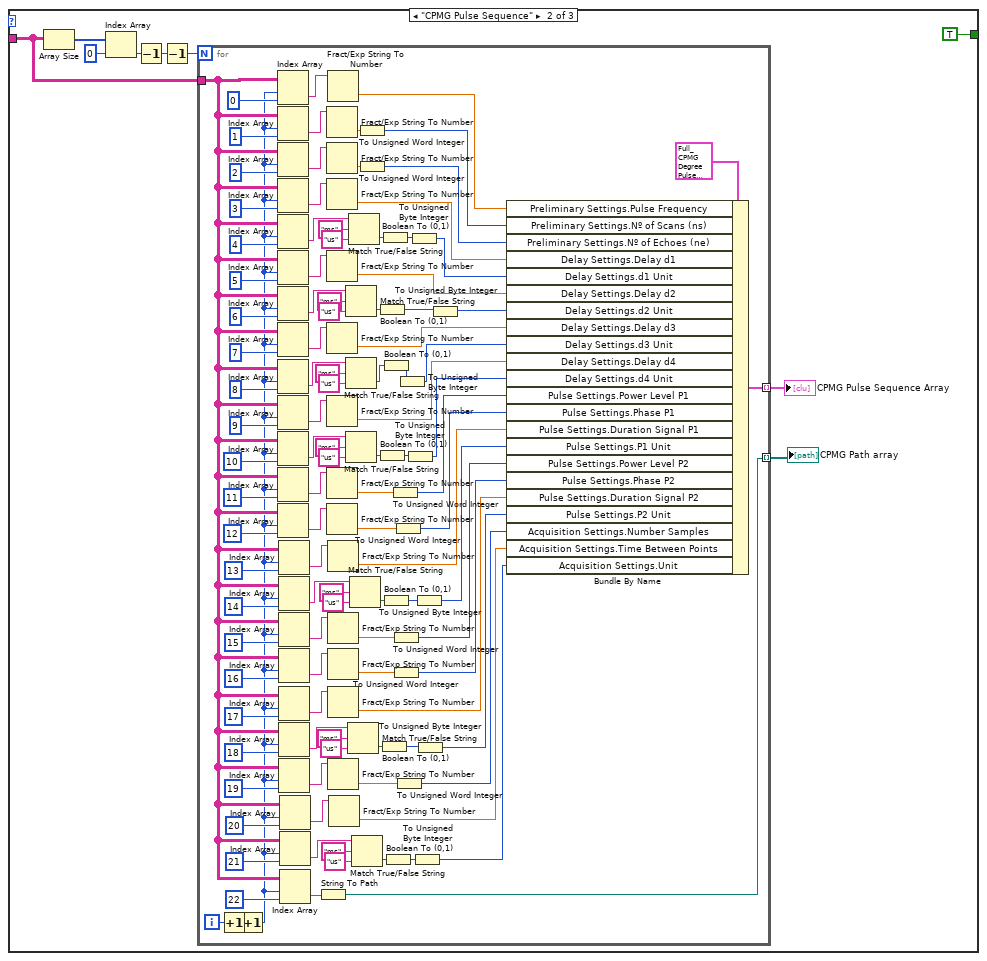
[diagram p3: hidden frame]
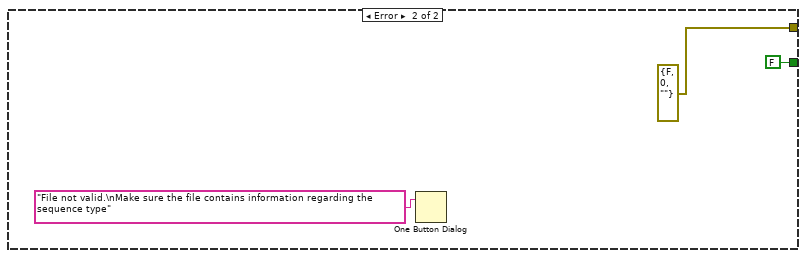
[diagram p4: hidden frame]
diagram:
  n1 = while {
    tunnel: [w4] -> w2
    tunnel: "error in (no error)" -> [w6]
    stop <- w14 stop-if-true
    n2 = call "File Dialog"("prompt"="Choose Loop file", "button label"="Done", "error in"=w6, "pattern (all files)"="*xlsx;" ("pattern")) -> ("selected path"=w9:path, "error out"=w8:errorcluster)  [unwired: 8 in, 2 out]
    n3 = call "XLS_to_TXT.vi"("error in (no error)"=w8, "Path"=w9) -> ("error out"=w7:errorcluster, "Path out"=w3:path)  [unwired: 8 in]
    n4 = call-poly <vilib>:"Read From Spreadsheet File.vi"("file path (dialog if empty)"=w3) -> ("first row"=w18:string[], "all rows"=w19:string[][])  [unwired: 6 in, 3 out]
    n5 = Index Array(array=w18, index=1) -> (element=w12:string)
    n6 = Scan From String(input string=w12, error in=w7, default 1=NMR_Pulse_Sequence_Type."90 Degree Sequence" ("Pulse Sequence Type")) -> (error out=w11:errorcluster, output 1=w10:T1)  [unwired: 2 in, 2 out]
    "Sequence Type" <- w10
    n7 = case shown="No Error" w11 {
      selector: w11 -> [w21 _]
      tunnel: w19 -> [w24 _]
      tunnel: [w23 FALSE] -> w14
      tunnel: w10 -> [w22 _]
      tunnel: [w21 errorcluster {"status"=FALSE, "code"=0, "source"=""} ("error IO")] -> w5
      frame No Error {
        n8 = case shown="\"T1 Pulse Sequence\"" w22 {
          tunnel: w24 -> [w29 w105 w224]
          tunnel: [TRUE TRUE TRUE] -> w23
          frame "90 Degree Sequence" {
            n9 = Array Size(array=w29) -> (size(s)=w30:i32[])
            n10 = Index Array(array=w30, index=0) -> (element=w32:i32)
            n11 = Decrement(x=w32) -> (x-1=w33:i32)
            n12 = Decrement(x=w33) -> (x-1=w28:i32)
            n13 = for {
              N: w28 -> [_]
              tunnel: w29 -> [w81]
              tunnel: [w55] -> w25 mode=indexing
              tunnel: [w54] -> w27 mode=indexing
              i -> [w94]
              n14 = Increment(x=w94) -> (x+1=w98:i32)
              n15 = Increment(x=w98) -> (x+1=w80:i32)
              n16 = Index Array(array=w81, index (row)=w80, index (col)=0) -> (element=w97:string)
              n17 = Index Array(array=w81, index (row)=w80, index (col)=1 ("index (row)")) -> (element=w96:string)
              n18 = Index Array(array=w81, index (row)=w80, index (col)=2 ("index (row)")) -> (element=w79:string)
              n19 = Index Array(array=w81, index (row)=w80, index (col)=3 ("index (row)")) -> (element=w43:string)
              n20 = Index Array(array=w81, index (row)=w80, index (col)=4 ("index (row)")) -> (element=w78:string)
              n21 = Index Array(array=w81, index (row)=w80, index (col)=5 ("index (row)")) -> (element=w42:string)
              n22 = Index Array(array=w81, index (row)=w80, index (col)=6 ("index (row)")) -> (element=w77:string)
              n23 = Index Array(array=w81, index (row)=w80, index (col)=7 ("index (row)")) -> (element=w76:string)
              n24 = Index Array(array=w81, index (row)=w80, index (col)=8 ("index (row)")) -> (element=w75:string)
              n25 = Index Array(array=w81, index (row)=w80, index (col)=9 ("index (row)")) -> (element=w41:string)
              n26 = Index Array(array=w81, index (row)=w80, index (col)=10 ("index (row)")) -> (element=w74:string)
              n27 = Index Array(array=w81, index (row)=w80, index (col)=11 ("index (row)")) -> (element=w73:string)
              n28 = Index Array(array=w81, index (row)=w80, index (col)=12 ("index (row)")) -> (element=w40:string)
              n29 = Index Array(array=w81, index (row)=w80, index (col)=13 ("index (row)")) -> (element=w95:string)
              n30 = String To Path(string=w95) -> (path=w54:path)
              n31 = Match True/False String(2:"us" ("true string"), 3:"ms" ("false string"), 4:w42) -> (0:w48:bool)  [unwired: 1 out]
              n32 = Fract/Exp String To Number(string=w96) -> (number=w70:dbl)  [unwired: 3 in, 1 out]
              n33 = Fract/Exp String To Number(string=w79) -> (number=w68:dbl)  [unwired: 3 in, 1 out]
              n34 = Match True/False String(2:"us" ("true string"), 3:"ms" ("false string"), 4:w43) -> (0:w53:bool)  [unwired: 1 out]
              n35 = Fract/Exp String To Number(string=w78) -> (number=w64:dbl)  [unwired: 3 in, 1 out]
              n36 = Fract/Exp String To Number(string=w77) -> (number=w63:dbl)  [unwired: 3 in, 1 out]
              n37 = Fract/Exp String To Number(string=w76) -> (number=w60:dbl)  [unwired: 3 in, 1 out]
              n38 = Fract/Exp String To Number(string=w75) -> (number=w59:dbl)  [unwired: 3 in, 1 out]
              n39 = Match True/False String(2:"us" ("true string"), 3:"ms" ("false string"), 4:w41) -> (0:w39:bool)  [unwired: 1 out]
              n40 = Fract/Exp String To Number(string=w74) -> (number=w56:dbl)  [unwired: 3 in, 1 out]
              n41 = Fract/Exp String To Number(string=w73) -> (number=w72:dbl)  [unwired: 3 in, 1 out]
              n42 = Match True/False String(2:"us" ("true string"), 3:"ms" ("false string"), 4:w40) -> (0:w38:bool)  [unwired: 1 out]
              n43 = Fract/Exp String To Number(string=w97) -> (number=w71:dbl)  [unwired: 3 in, 1 out]
              n44 = Boolean To (0,1)(Boolean=w48) -> (0, 1=w35:i16)
              n45 = Boolean To (0,1)(Boolean=w53) -> (0, 1=w34:i16)
              n46 = Boolean To (0,1)(Boolean=w39) -> (0, 1=w36:i16)
              n47 = Boolean To (0,1)(Boolean=w38) -> (0, 1=w37:i16)
              n48 = To Unsigned Word Integer(number=w70) -> (unsigned 16bit integer=w69:u16)
              n49 = To Unsigned Byte Integer(number=w34) -> (unsigned 8bit integer=w67:u8)
              n50 = To Unsigned Byte Integer(number=w36) -> (unsigned 8bit integer=w66:u8)
              n51 = To Unsigned Byte Integer(number=w35) -> (unsigned 8bit integer=w65:u8)
              n52 = To Unsigned Word Integer(number=w63) -> (unsigned 16bit integer=w62:u16)
              n53 = To Unsigned Word Integer(number=w56) -> (unsigned 16bit integer=w57:u16)
              n54 = To Unsigned Word Integer(number=w60) -> (unsigned 16bit integer=w61:u16)
              n55 = To Unsigned Byte Integer(number=w37) -> (unsigned 8bit integer=w58:u8)
              n56 = Bundle By Name(cluster=T11 {"Delay Settings"={"Delay d1"=10.0, "Delay d2"=0.0, "d1 Unit"=0, "d2 Unit"=0}, "Preliminary Settings"={"Nº of Scans (ns)"=3, "Pulse Frequency"=10000000.0}, "Pulse Settings"={"Duration Signal P1"=20.0, "Power Level"=1023, "Phase"=90, "P1 Units"=0}, "Acquisition Settings"={"Number Samples"=2000, "Time Between Points"=0.0, "Unit"=0}} ("90 Degree Pulse Sequence 2"), "Preliminary Settings.Pulse Frequency"=w71, "Preliminary Settings.Nº of Scans (ns)"=w69, "Delay Settings.Delay d1"=w68, "Delay Settings.d1 Unit"=w67, "Delay Settings.Delay d2"=w64, "Delay Settings.d2 Unit"=w65, "Pulse Settings.Power Level"=w62, "Pulse Settings.Phase"=w61, "Pulse Settings.Duration Signal P1"=w59, "Pulse Settings.P1 Units"=w66, "Acquisition Settings.Number Samples"=w57, "Acquisition Settings.Time Between Points"=w72, "Acquisition Settings.Unit"=w58) -> (w55:T11)
            }
            "90Deg Pulse Sequence Array" <- w25
            "90Deg path array" <- w27
          }
          frame "CPMG Pulse Sequence" {
            n57 = Array Size(array=w105) -> (size(s)=w107:i32[])
            n58 = Index Array(array=w107, index=0) -> (element=w109:i32)
            n59 = Decrement(x=w109) -> (x-1=w110:i32)
            n60 = Decrement(x=w110) -> (x-1=w106:i32)
            n61 = for {
              N: w106 -> [_]
              tunnel: w105 -> [w160]
              tunnel: [w147] -> w104 mode=indexing
              tunnel: [w146] -> w103 mode=indexing
              i -> [w213]
              n62 = Increment(x=w213) -> (x+1=w217:i32)
              n63 = Increment(x=w217) -> (x+1=w151:i32)
              n64 = Index Array(array=w160, index (row)=w151, index (col)=0) -> (element=w216:string)
              n65 = Index Array(array=w160, index (row)=w151, index (col)=1 ("index (row)")) -> (element=w215:string)
              n66 = Index Array(array=w160, index (row)=w151, index (col)=2 ("index (row)")) -> (element=w201:string)
              n67 = Index Array(array=w160, index (row)=w151, index (col)=3 ("index (row)")) -> (element=w200:string)
              n68 = Index Array(array=w160, index (row)=w151, index (col)=4 ("index (row)")) -> (element=w141:string)
              n69 = Index Array(array=w160, index (row)=w151, index (col)=5 ("index (row)")) -> (element=w199:string)
              n70 = Index Array(array=w160, index (row)=w151, index (col)=6 ("index (row)")) -> (element=w136:string)
              n71 = Index Array(array=w160, index (row)=w151, index (col)=7 ("index (row)")) -> (element=w198:string)
              n72 = Index Array(array=w160, index (row)=w151, index (col)=8 ("index (row)")) -> (element=w131:string)
              n73 = Index Array(array=w160, index (row)=w151, index (col)=9 ("index (row)")) -> (element=w197:string)
              n74 = Index Array(array=w160, index (row)=w151, index (col)=10 ("index (row)")) -> (element=w126:string)
              n75 = Index Array(array=w160, index (row)=w151, index (col)=11 ("index (row)")) -> (element=w196:string)
              n76 = Index Array(array=w160, index (row)=w151, index (col)=12 ("index (row)")) -> (element=w195:string)
              n77 = Index Array(array=w160, index (row)=w151, index (col)=13 ("index (row)")) -> (element=w173:string)
              n78 = Index Array(array=w160, index (row)=w151, index (col)=14 ("index (row)")) -> (element=w121:string)
              n79 = Index Array(array=w160, index (row)=w151, index (col)=15 ("index (row)")) -> (element=w174:string)
              n80 = Index Array(array=w160, index (row)=w151, index (col)=16 ("index (row)")) -> (element=w175:string)
              n81 = Index Array(array=w160, index (row)=w151, index (col)=17 ("index (row)")) -> (element=w148:string)
              n82 = Index Array(array=w160, index (row)=w151, index (col)=18 ("index (row)")) -> (element=w116:string)
              n83 = Index Array(array=w160, index (row)=w151, index (col)=19 ("index (row)")) -> (element=w164:string)
              n84 = Index Array(array=w160, index (row)=w151, index (col)=20 ("index (row)")) -> (element=w166:string)
              n85 = Index Array(array=w160, index (row)=w151, index (col)=21 ("index (row)")) -> (element=w111:string)
              n86 = Index Array(array=w160, index (row)=w151, index (col)=22 ("index (row)")) -> (element=w214:string)
              n87 = String To Path(string=w214) -> (path=w146:path)
              n88 = Fract/Exp String To Number(string=w215) -> (number=w193:dbl)  [unwired: 3 in, 1 out]
              n89 = Fract/Exp String To Number(string=w201) -> (number=w189:dbl)  [unwired: 3 in, 1 out]
              n90 = Fract/Exp String To Number(string=w200) -> (number=w188:dbl)  [unwired: 3 in, 1 out]
              n91 = Fract/Exp String To Number(string=w199) -> (number=w186:dbl)  [unwired: 3 in, 1 out]
              n92 = Fract/Exp String To Number(string=w198) -> (number=w184:dbl)  [unwired: 3 in, 1 out]
              n93 = Fract/Exp String To Number(string=w197) -> (number=w182:dbl)  [unwired: 3 in, 1 out]
              n94 = Fract/Exp String To Number(string=w196) -> (number=w180:dbl)  [unwired: 3 in, 1 out]
              n95 = Fract/Exp String To Number(string=w195) -> (number=w178:dbl)  [unwired: 3 in, 1 out]
              n96 = Fract/Exp String To Number(string=w216) -> (number=w194:dbl)  [unwired: 3 in, 1 out]
              n97 = Fract/Exp String To Number(string=w173) -> (number=w159:dbl)  [unwired: 3 in, 1 out]
              n98 = Fract/Exp String To Number(string=w174) -> (number=w176:dbl)  [unwired: 3 in, 1 out]
              n99 = Fract/Exp String To Number(string=w175) -> (number=w156:dbl)  [unwired: 3 in, 1 out]
              n100 = Fract/Exp String To Number(string=w148) -> (number=w154:dbl)  [unwired: 3 in, 1 out]
              n101 = Fract/Exp String To Number(string=w164) -> (number=w165:dbl)  [unwired: 3 in, 1 out]
              n102 = Fract/Exp String To Number(string=w166) -> (number=w150:dbl)  [unwired: 3 in, 1 out]
              n103 = Match True/False String(2:"us" ("true string"), 3:"ms" ("false string"), 4:w136) -> (0:w138:bool)  [unwired: 1 out]
              n104 = Match True/False String(2:"us" ("true string"), 3:"ms" ("false string"), 4:w131) -> (0:w133:bool)  [unwired: 1 out]
              n105 = Match True/False String(2:"us" ("true string"), 3:"ms" ("false string"), 4:w126) -> (0:w128:bool)  [unwired: 1 out]
              n106 = Match True/False String(2:"us" ("true string"), 3:"ms" ("false string"), 4:w116) -> (0:w118:bool)  [unwired: 1 out]
              n107 = Match True/False String(2:"us" ("true string"), 3:"ms" ("false string"), 4:w141) -> (0:w145:bool)  [unwired: 1 out]
              n108 = Match True/False String(2:"us" ("true string"), 3:"ms" ("false string"), 4:w121) -> (0:w123:bool)  [unwired: 1 out]
              n109 = Match True/False String(2:"us" ("true string"), 3:"ms" ("false string"), 4:w111) -> (0:w113:bool)  [unwired: 1 out]
              n110 = To Unsigned Word Integer(number=w193) -> (unsigned 16bit integer=w192:u16)
              n111 = To Unsigned Word Integer(number=w189) -> (unsigned 16bit integer=w190:u16)
              n112 = Boolean To (0,1)(Boolean=w138) -> (0, 1=w137:i16)
              n113 = Boolean To (0,1)(Boolean=w128) -> (0, 1=w127:i16)
              n114 = Boolean To (0,1)(Boolean=w118) -> (0, 1=w117:i16)
              n115 = Boolean To (0,1)(Boolean=w145) -> (0, 1=w142:i16)
              n116 = Boolean To (0,1)(Boolean=w133) -> (0, 1=w132:i16)
              n117 = Boolean To (0,1)(Boolean=w123) -> (0, 1=w122:i16)
              n118 = Boolean To (0,1)(Boolean=w113) -> (0, 1=w112:i16)
              n119 = To Unsigned Word Integer(number=w180) -> (unsigned 16bit integer=w179:u16)
              n120 = To Unsigned Word Integer(number=w176) -> (unsigned 16bit integer=w157:u16)
              n121 = To Unsigned Word Integer(number=w156) -> (unsigned 16bit integer=w155:u16)
              n122 = To Unsigned Word Integer(number=w178) -> (unsigned 16bit integer=w177:u16)
              n123 = To Unsigned Word Integer(number=w165) -> (unsigned 16bit integer=w152:u16)
              n124 = To Unsigned Byte Integer(number=w132) -> (unsigned 8bit integer=w183:u8)
              n125 = To Unsigned Byte Integer(number=w127) -> (unsigned 8bit integer=w181:u8)
              n126 = To Unsigned Byte Integer(number=w142) -> (unsigned 8bit integer=w187:u8)
              n127 = To Unsigned Byte Integer(number=w112) -> (unsigned 8bit integer=w149:u8)
              n128 = To Unsigned Byte Integer(number=w122) -> (unsigned 8bit integer=w158:u8)
              n129 = To Unsigned Byte Integer(number=w117) -> (unsigned 8bit integer=w153:u8)
              n130 = To Unsigned Byte Integer(number=w137) -> (unsigned 8bit integer=w185:u8)
              n131 = Bundle By Name(cluster=T7 {"Acquisition Settings"={"Number Samples"=2000, "Time Between Points"=0.0, "Unit"=0}, "Delay Settings"={"Delay d1"=10.0, "Delay d2"=0.0, "d1 Unit"=0, "d2 Unit"=0, "Delay d3"=0.0, "d3 Unit"=0, "Delay d4"=0.0, "d4 Unit"=0}, "Preliminary Settings"={"Nº of Scans (ns)"=3, "Pulse Frequency"=10000000.0, "Nº of Echoes (ne)"=3}, "Pulse Settings"={"Duration Signal P1"=20.0, "Power Level P1"=1023, "Phase P1"=90, "P1 Unit"=0, "Duration Signal P2"=20.0, "Power Level P2"=1023, "Phase P2"=90, "P2 Unit"=0}} ("CPMG Pulse Sequence 2"), "Preliminary Settings.Pulse Frequency"=w194, "Preliminary Settings.Nº of Scans (ns)"=w192, "Preliminary Settings.Nº of Echoes (ne)"=w190, "Delay Settings.Delay d1"=w188, "Delay Settings.d1 Unit"=w187, "Delay Settings.Delay d2"=w186, "Delay Settings.d2 Unit"=w185, "Delay Settings.Delay d3"=w184, "Delay Settings.d3 Unit"=w183, "Delay Settings.Delay d4"=w182, "Delay Settings.d4 Unit"=w181, "Pulse Settings.Power Level P1"=w179, "Pulse Settings.Phase P1"=w177, "Pulse Settings.Duration Signal P1"=w159, "Pulse Settings.P1 Unit"=w158, "Pulse Settings.Power Level P2"=w157, "Pulse Settings.Phase P2"=w155, "Pulse Settings.Duration Signal P2"=w154, "Pulse Settings.P2 Unit"=w153, "Acquisition Settings.Number Samples"=w152, "Acquisition Settings.Time Between Points"=w150, "Acquisition Settings.Unit"=w149) -> (w147:T7)
            }
            "CPMG Pulse Sequence Array" <- w104
            "CPMG Path array" <- w103
          }
          frame "T1 Pulse Sequence" {
            n132 = Array Size(array=w224) -> (size(s)=w226:i32[])
            n133 = Index Array(array=w226, index=0) -> (element=w228:i32)
            n134 = Decrement(x=w228) -> (x-1=w229:i32)
            n135 = Decrement(x=w229) -> (x-1=w225:i32)
            n136 = for {
              N: w225 -> [_]
              tunnel: w224 -> [w275]
              tunnel: [w256] -> w223 mode=indexing
              tunnel: [w255] -> w222 mode=indexing
              i -> [w316]
              n137 = Increment(x=w316) -> (x+1=w320:i32)
              n138 = Increment(x=w320) -> (x+1=w257:i32)
              n139 = Index Array(array=w275, index (row)=w257, index (col)=0) -> (element=w319:string)
              n140 = Index Array(array=w275, index (row)=w257, index (col)=1 ("index (row)")) -> (element=w318:string)
              n141 = Index Array(array=w275, index (row)=w257, index (col)=2 ("index (row)")) -> (element=w308:string)
              n142 = Index Array(array=w275, index (row)=w257, index (col)=3 ("index (row)")) -> (element=w307:string)
              n143 = Index Array(array=w275, index (row)=w257, index (col)=4 ("index (row)")) -> (element=w250:string)
              n144 = Index Array(array=w275, index (row)=w257, index (col)=5 ("index (row)")) -> (element=w306:string)
              n145 = Index Array(array=w275, index (row)=w257, index (col)=6 ("index (row)")) -> (element=w245:string)
              n146 = Index Array(array=w275, index (row)=w257, index (col)=7 ("index (row)")) -> (element=w305:string)
              n147 = Index Array(array=w275, index (row)=w257, index (col)=8 ("index (row)")) -> (element=w304:string)
              n148 = Index Array(array=w275, index (row)=w257, index (col)=9 ("index (row)")) -> (element=w288:string)
              n149 = Index Array(array=w275, index (row)=w257, index (col)=10 ("index (row)")) -> (element=w240:string)
              n150 = Index Array(array=w275, index (row)=w257, index (col)=11 ("index (row)")) -> (element=w289:string)
              n151 = Index Array(array=w275, index (row)=w257, index (col)=12 ("index (row)")) -> (element=w290:string)
              n152 = Index Array(array=w275, index (row)=w257, index (col)=13 ("index (row)")) -> (element=w264:string)
              n153 = Index Array(array=w275, index (row)=w257, index (col)=14 ("index (row)")) -> (element=w236:string)
              n154 = Index Array(array=w275, index (row)=w257, index (col)=15 ("index (row)")) -> (element=w279:string)
              n155 = Index Array(array=w275, index (row)=w257, index (col)=16 ("index (row)")) -> (element=w281:string)
              n156 = Index Array(array=w275, index (row)=w257, index (col)=17 ("index (row)")) -> (element=w231:string)
              n157 = Index Array(array=w275, index (row)=w257, index (col)=18 ("index (row)")) -> (element=w317:string)
              n158 = String To Path(string=w317) -> (path=w255:path)
              n159 = Fract/Exp String To Number(string=w318) -> (number=w302:dbl)  [unwired: 3 in, 1 out]
              n160 = Fract/Exp String To Number(string=w308) -> (number=w300:dbl)  [unwired: 3 in, 1 out]
              n161 = Fract/Exp String To Number(string=w307) -> (number=w299:dbl)  [unwired: 3 in, 1 out]
              n162 = Fract/Exp String To Number(string=w306) -> (number=w297:dbl)  [unwired: 3 in, 1 out]
              n163 = Fract/Exp String To Number(string=w305) -> (number=w295:dbl)  [unwired: 3 in, 1 out]
              n164 = Fract/Exp String To Number(string=w304) -> (number=w293:dbl)  [unwired: 3 in, 1 out]
              n165 = Fract/Exp String To Number(string=w319) -> (number=w303:dbl)  [unwired: 3 in, 1 out]
              n166 = Fract/Exp String To Number(string=w288) -> (number=w274:dbl)  [unwired: 3 in, 1 out]
              n167 = Fract/Exp String To Number(string=w289) -> (number=w291:dbl)  [unwired: 3 in, 1 out]
              n168 = Fract/Exp String To Number(string=w290) -> (number=w271:dbl)  [unwired: 3 in, 1 out]
              n169 = Fract/Exp String To Number(string=w264) -> (number=w269:dbl)  [unwired: 3 in, 1 out]
              n170 = Fract/Exp String To Number(string=w279) -> (number=w280:dbl)  [unwired: 3 in, 1 out]
              n171 = Fract/Exp String To Number(string=w281) -> (number=w266:dbl)  [unwired: 3 in, 1 out]
              n172 = Match True/False String(2:"us" ("true string"), 3:"ms" ("false string"), 4:w250) -> (0:w254:bool)  [unwired: 1 out]
              n173 = Match True/False String(2:"us" ("true string"), 3:"ms" ("false string"), 4:w240) -> (0:w244:bool)  [unwired: 1 out]
              n174 = Match True/False String(2:"us" ("true string"), 3:"ms" ("false string"), 4:w236) -> (0:w237:bool)  [unwired: 1 out]
              n175 = Match True/False String(2:"us" ("true string"), 3:"ms" ("false string"), 4:w245) -> (0:w247:bool)  [unwired: 1 out]
              n176 = Match True/False String(2:"us" ("true string"), 3:"ms" ("false string"), 4:w231) -> (0:w234:bool)  [unwired: 1 out]
              n177 = To Unsigned Word Integer(number=w295) -> (unsigned 16bit integer=w294:u16)
              n178 = Boolean To (0,1)(Boolean=w254) -> (0, 1=w251:i16)
              n179 = To Unsigned Word Integer(number=w291) -> (unsigned 16bit integer=w272:u16)
              n180 = To Unsigned Word Integer(number=w271) -> (unsigned 16bit integer=w270:u16)
              n181 = To Unsigned Word Integer(number=w293) -> (unsigned 16bit integer=w292:u16)
              n182 = Boolean To (0,1)(Boolean=w244) -> (0, 1=w241:i16)
              n183 = To Unsigned Word Integer(number=w280) -> (unsigned 16bit integer=w267:u16)
              n184 = Boolean To (0,1)(Boolean=w237) -> (0, 1=w235:i16)
              n185 = Boolean To (0,1)(Boolean=w247) -> (0, 1=w246:i16)
              n186 = Boolean To (0,1)(Boolean=w234) -> (0, 1=w230:i16)
              n187 = To Unsigned Word Integer(number=w302) -> (unsigned 16bit integer=w301:u16)
              n188 = To Unsigned Word Integer(number=w300) -> (unsigned 16bit integer=w262:u16)
              n189 = To Unsigned Byte Integer(number=w251) -> (unsigned 8bit integer=w298:u8)
              n190 = To Unsigned Byte Integer(number=w241) -> (unsigned 8bit integer=w273:u8)
              n191 = To Unsigned Byte Integer(number=w246) -> (unsigned 8bit integer=w296:u8)
              n192 = To Unsigned Byte Integer(number=w235) -> (unsigned 8bit integer=w268:u8)
              n193 = To Unsigned Byte Integer(number=w230) -> (unsigned 8bit integer=w265:u8)
              n194 = Bundle By Name(cluster=T2 {"Preliminary Settings"={"Nº of Scans (ns)"=3, "Pulse Frequency"=10000000.0, "Nº of Vd"=3}, "Pulse Settings"={"Duration Signal P2"=20.0, "Power Level P2"=1023, "Phase P2"=90, "P2 Unit"=0, "Duration Signal P1"=20.0, "Power Level P1"=1023, "Phase P1"=90, "P1 Unit"=0}, "Acquisition Settings"={"Number Samples"=2000, "Time Between Points"=0.0, "Unit"=0}, "Delay Settings"={"Delay d1"=10.0, "Delay d2"=0.0, "d1 Unit"=0, "d2 Unit"=0, "Delay d30"=0.0, "d30 Unit"=0, "Vd Unit"=0, "Vd Values"="0"}} ("T1 Pulse Sequence 2"), "Preliminary Settings.Pulse Frequency"=w303, "Preliminary Settings.Nº of Scans (ns)"=w301, "Preliminary Settings.Nº of Vd"=w262, "Delay Settings.Delay d1"=w299, "Delay Settings.d1 Unit"=w298, "Delay Settings.Delay d2"=w297, "Delay Settings.d2 Unit"=w296, "Delay Settings.Delay d30"=0.0, "Delay Settings.d30 Unit"=u8 0, "Delay Settings.Vd Values"="Automatic", "Delay Settings.Vd Unit"=u8 0, "Pulse Settings.Power Level P2"=w294, "Pulse Settings.Phase P2"=w292, "Pulse Settings.Duration Signal P2"=w274, "Pulse Settings.P2 Unit"=w273, "Pulse Settings.Power Level P1"=w272, "Pulse Settings.Phase P1"=w270, "Pulse Settings.Duration Signal P1"=w269, "Pulse Settings.P1 Unit"=w268, "Acquisition Settings.Number Samples"=w267, "Acquisition Settings.Time Between Points"=w266, "Acquisition Settings.Unit"=w265) -> (w256:T2)
            }
            "T1 Pulse Sequence Array" <- w223
            "T1 path array" <- w222
          }
        }
      }
      frame Error {
        n195 = One Button Dialog(message="File not valid.\nMake sure the file contains information regarding the  sequence type") -> ()  [unwired: 1 in, 1 out]
      }
    }
    n196 = Delete(path (use dialog)=w3, error in=w5) -> (error out=w4:errorcluster)  [unwired: 3 in, 2 out]
  }
  "error out" <- w2
